vi "sub_Loop.vi"(0 "Input parameters":T2={"Measurement type"=enum."Test", "Sensor type"=enum."One channel", "Input file"="", "Output file"="test.txt", "Open after execution?"=FALSE, "Display channel"=0, "Voltage Delay (s)"=0.5, "Switch Delay (s)"=0.01, "VISA resource name source"="", "VISA resource name LCR"="", "Voltage Limit (V)"=1000.0, "Enable Voltage Auto Range (T:Enable)"=TRUE, "Voltage Manual Range (1.0)"=1.0, "Compliance  Level (uA)"=10.0} {"Voltage Limit (V)" format="%#_13g"; "Voltage Delay (s)" format="%#_13g"; "Switch Delay (s)" format="%#_13g"}, 2 "Current voltage":refnum<vi>, 3 "Voltages":refnum<vi>, 5 "Dynamic data 2":T1, 8 "Channels":refnum<vi>, 9 "Stop":refnum<vi>, 10 "Single channel":refnum<vi>, 11 "error in (no error)":errorcluster, 13 "Current channel":refnum<vi>) -> (4 "Input parameters":T2={"Measurement type"=enum."Test", "Sensor type"=enum."One channel", "Input file"="", "Output file"="test.txt", "Open after execution?"=FALSE, "Display channel"=0, "Voltage Delay (s)"=0.5, "Switch Delay (s)"=0.01, "VISA resource name source"="", "VISA resource name LCR"="", "Voltage Limit (V)"=1000.0, "Enable Voltage Auto Range (T:Enable)"=TRUE, "Voltage Manual Range (1.0)"=1.0, "Compliance  Level (uA)"=10.0} {"Voltage Limit (V)" format="%#_13g"; "Voltage Delay (s)" format="%#_13g"; "Switch Delay (s)" format="%#_13g"}, 6 "Dynamic data":T1, 15 "error out":errorcluster)   [LabVIEW 2015]
uses:
  Program Files (x86)/National Instruments/LabVIEW 2016/instr.lib/Keithley 24XX/Keithley 24XX.lvlib
  Program Files (x86)/National Instruments/LabVIEW 2016/instr.lib/Agilent 428X Series/Agilent 428X Series.lvlib
  Program Files (x86)/National Instruments/LabVIEW 2016/instr.lib/Keithley 24XX/Public/Data/Read (Single Point).vi
  Input_parameters.ctl
  Dynamic_data.ctl
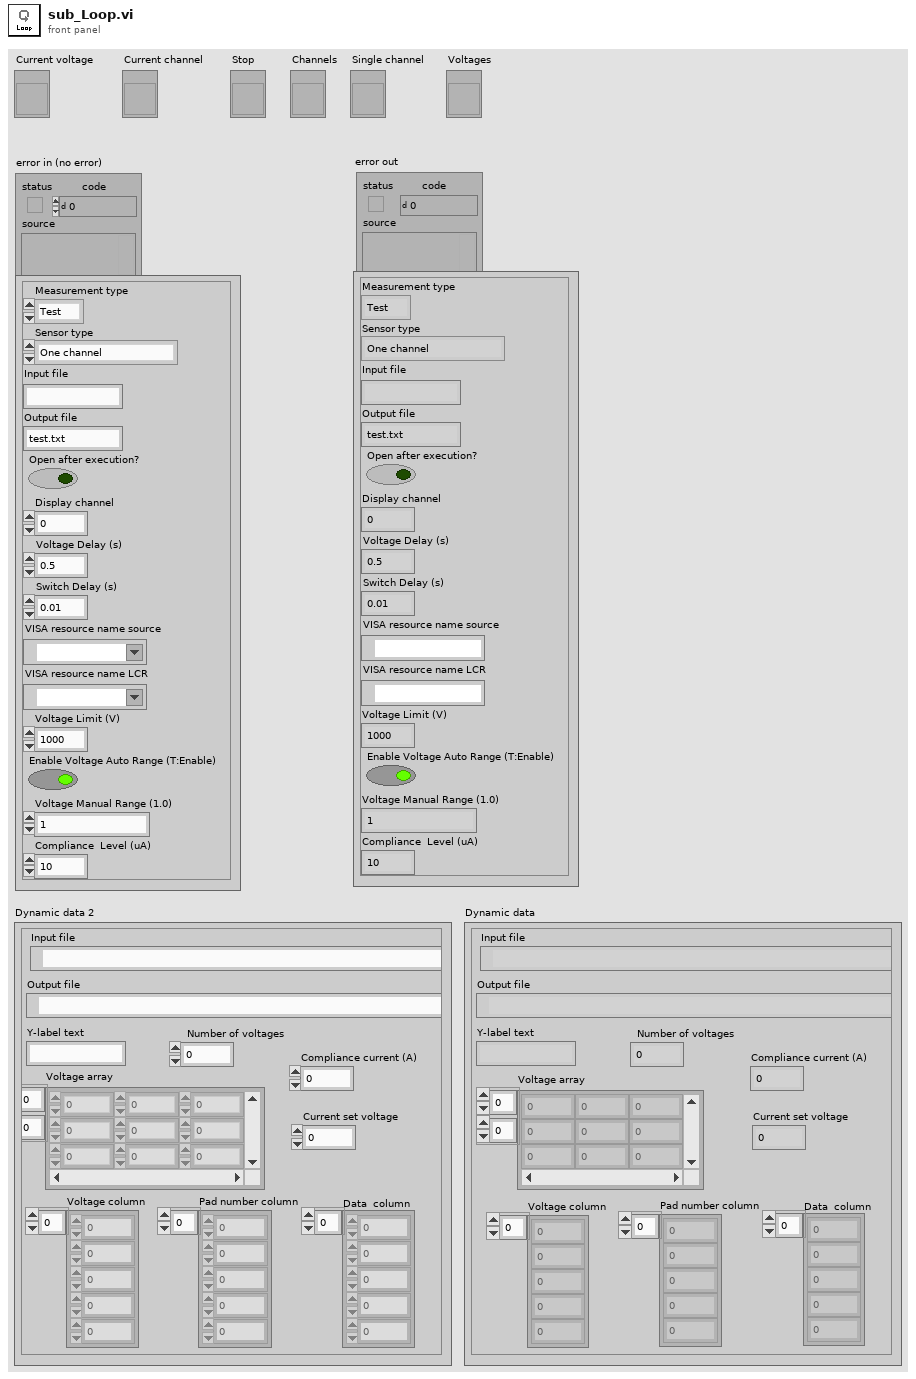
[diagram p1: front panel]
types:
  T1 = typedef "Dynamic_data.ctl" = cluster{"Input file":path, "Output file":path, "Y-label text":string, "Voltage array":dbl[][], "Current set voltage":dbl, "Voltage column":dbl[], "Pad number column":dbl[], "Data  column":dbl[], "Number of voltages":i32, "Compliance current (A)":dbl}
  T2 = typedef "Input_parameters.ctl" = cluster{"Measurement type":enum16{"IV", "CV", "Test"}, "Sensor type":enum16{"6''", "8''", "One channel"}, "Input file":string, "Output file":string, "Open after execution?":bool, "Display channel":i32, "Voltage Delay (s)":dbl, "Switch Delay (s)":dbl, "VISA resource name source":refnum<visa-resource-name>, "VISA resource name LCR":refnum<visa-resource-name>, "Voltage Limit (V)":dbl, "Enable Voltage Auto Range (T:Enable)":bool, "Voltage Manual Range (1.0)":dbl, "Compliance  Level (uA)":dbl}
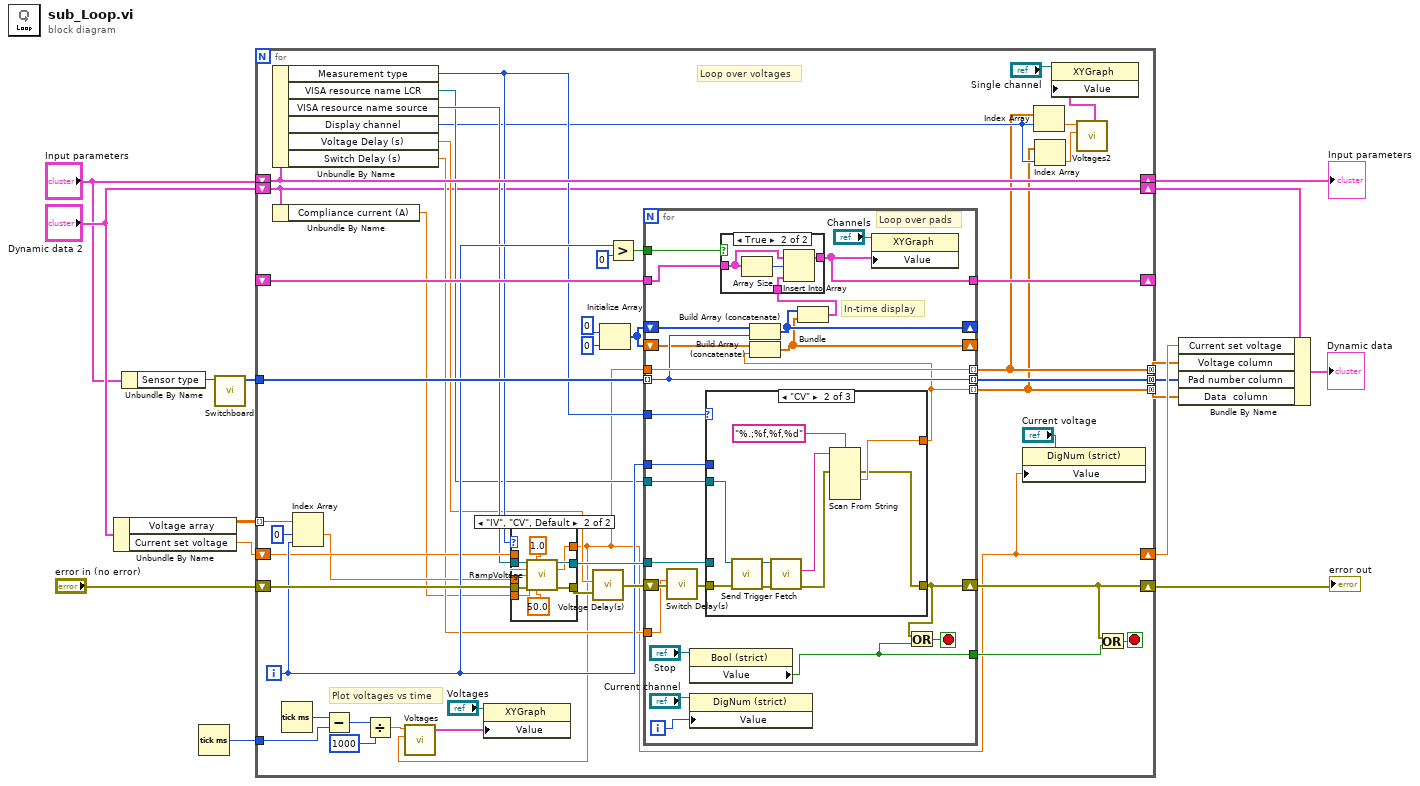
[diagram p0: block diagram]
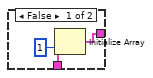
[diagram p3: hidden frame]
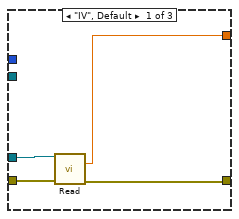
[diagram p4: hidden frame]
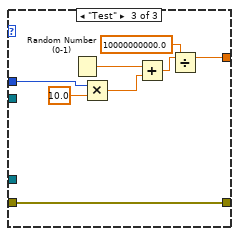
[diagram p5: hidden frame]
diagram:
  n1 = Unbundle By Name("Dynamic data 2") -> ("Voltage array"=w15:dbl[][], "Current set voltage"=w13:dbl)
  n2 = Unbundle By Name("Input parameters") -> ("Sensor type"=w16:enum16{"6''", "8''", "One channel"})
  n3 = Tick Count (ms)() -> (millisecond timer value=w1:u32)
  n4 = call "Switchboard.vi"("Sensor type"=w16) -> ("Output config"=w14:i32[])  [unwired: 10 in]
  n5 = for {
    tunnel: w15 -> [w61] mode=indexing
    tunnel: w14 -> [w59]
    tunnel: [w22] -> w11 mode=concatenating
    tunnel: [w21] -> w9 mode=concatenating
    tunnel: [w57] -> w10 mode=concatenating
    shift-right: [w43] -> w2
    shift-left: "error in (no error)" -> [w55]
    shift-right: [w51] -> _
    shift-left: _ -> [w50]
    shift-right: [w26] -> w12
    shift-left: w13 -> [w42]
    shift-right: [w40] -> w4
    shift-left: "Input parameters" -> [w40]
    shift-right: [w34] -> w8
    shift-left: "Dynamic data 2" -> [w34]
    tunnel: w1 -> [w27]
    i -> [w46]
    stop <- w44 stop-if-true
    # "Plot voltages vs time"
    # "Loop over voltages"
    n6 = Unbundle By Name(w40) -> ("Measurement type"=w39:enum16{"IV", "CV", "Test"}, "VISA resource name LCR"=w37:refnum<visa-resource-name>, "VISA resource name source"=w38:refnum<visa-resource-name>, "Display channel"=w23:i32, "Voltage Delay (s)"=w36:dbl, "Switch Delay (s)"=w35:dbl)
    n7 = Unbundle By Name(w34) -> ("Compliance current (A)"=w33:dbl)
    n8 = Tick Count (ms)() -> (millisecond timer value=w31:u32)
    n9 = Index Array(array=w61, index #1=0 ("index"), index #2=w46) -> (element #1=w41:dbl)  [unwired: 1 out]
    n10 = Subtract(x=w31, y=w27) -> (x-y=w30:u32)
    n11 = Divide(x=w30, y=u32 1000 ("x")) -> (x/y=w29:dbl)
    n12 = case shown="\"IV\", \"CV\", Default" w39 {
      tunnel: w38 -> [w64 w71]
      tunnel: w41 -> [w62 w70]
      tunnel: [w64 w73] -> w56
      tunnel: w55 -> [w63 w72]
      tunnel: [w63 w74] -> w54
      tunnel: w33 -> [_ w68]
      tunnel: w42 -> [_ w69]
      tunnel: [w62 w65] -> w26
      frame "Test" {
      }
      frame "IV", "CV", Default {
        n13 = call "RampVoltage.vi"("VISA resource name"=w71, "Delay (s)"=1.0, "Current voltage (V)"=w69, "Target voltage (V)"=w70, "Compliance Current (A)"=w68, "error in (no error)"=w72, "Step size (V)"=50.0) -> ("VISA resource name out"=w73:refnum<visa-resource-name>, "Current voltage out (V)"=w65:dbl, "error out"=w74:errorcluster)  [unwired: 6 in]
      }
    }
    n14 = call "Voltages"("Y Input"=w26, "X Input"=w29) -> ("XY Graph"=w17:cluster{"X":dbl[], "Y":dbl[]}[])  [unwired: 8 in, 1 out]
    n15 = property class="XYGraph"(reference="Voltages", "Value"=w17) -> ()  [unwired: 1 in, 2 out]
    n16 = call "Voltage Delay(s)"("error in (no error)"=w54, "Delay Time (s)"=w36) -> ("error out"=w53:errorcluster)  [unwired: 9 in]
    n17 = Initialize Array(0 ("dimension size"), 0 ("dimension size")) -> (w47:i32[])
    n18 = Greater?(x=w46, y=0) -> (0:w52:bool)
    n19 = for {
      tunnel: w59 -> [w95] mode=indexing
      tunnel: [w95] -> w57 mode=indexing
      tunnel: [w93] -> w21 mode=indexing
      tunnel: w26 -> [w99]
      tunnel: [w99] -> w22 mode=indexing
      tunnel: w56 -> [w97]
      tunnel: w39 -> [w98]
      shift-right: [w83] -> w43
      shift-left: w53 -> [w84]
      tunnel: w37 -> [w96]
      shift-right: [w91] -> _
      shift-left: w47 -> [w94]
      shift-right: [w90] -> _
      shift-left: w47 -> [w92]
      tunnel: w52 -> [w88]
      tunnel: w46 -> [w89]
      tunnel: w50 -> [w87]
      tunnel: [w75] -> w51
      tunnel: [w77] -> w45
      tunnel: w35 -> [w81]
      i -> [w79]
      stop <- w82 stop-if-true
      # "In-time display"
      # "Loop over pads"
      n20 = call "Switch Delay(s)"("error in (no error)"=w84, "Delay Time (s)"=w81) -> ("error out"=w85:errorcluster)  [unwired: 9 in]
      n21 = property class="Bool (strict)"(reference="Stop") -> ("Value"=w77:bool)  [unwired: 1 in, 2 out]
      n22 = property on="Property Node" class="DigNum (strict)"(reference="Current channel", "Value"=w79) -> ()  [unwired: 1 in, 2 out]
      n23 = case shown="\"CV\"" w98 {
        tunnel: [w110 w113 w121] -> w93
        tunnel: w97 -> [w108 _ _]
        tunnel: w85 -> [w109 w116 w127]
        tunnel: [w107 w111 w127] -> w83
        tunnel: w96 -> [_ w117 _]
        tunnel: w89 -> [_ _ w122]
        frame "IV", Default {
          n24 = call-poly "Read.vi"("VISA resource name"=w108, "error in (no error)"=w109) -> ("Current"=w110:sgl, "error out"=w107:errorcluster)  [unwired: 7 in, 5 out]
        }
        frame "CV" {
          n25 = call "Send Trigger.vi"("error in (no error)"=w116, "VISA resource name"=w117) -> ("error out"=w118:errorcluster, "VISA resource name out"=w119:refnum<visa-resource-name>)  [unwired: 8 in]
          n26 = call "Fetch.vi"("error in (no error)"=w118, "VISA resource name"=w119) -> ("error out"=w112:errorcluster, "Returned Data"=w114:string)  [unwired: 7 in, 1 out]
          n27 = Scan From String(format string="%.;%f,%f,%d", input string=w114, error in=w112) -> (error out=w111:errorcluster, output 1=w113:dbl)  [unwired: 6 in, 2 out]
        }
        frame "Test" {
          n28 = Random Number (0-1)() -> (number: 0 to 1=w126:dbl)
          n29 = Multiply(x=w122, y=10.0) -> (x*y=w123:dbl)
          n30 = Add(x=w126, y=w123) -> (x+y=w125:dbl)
          n31 = Divide(x=w125, y=10000000000.0) -> (x/y=w121:dbl)
        }
      }
      n32 = Build Array (concatenate)(w94, w95) -> (w91:i32[])
      n33 = Build Array (concatenate)(w92, w93) -> (w90:dbl[])
      n34 = Bundle(w91, w90) -> (w86:cluster{i32[], dbl[]})  [unwired: 1 out]
      n35 = case shown="True" w88 {
        tunnel: w87 -> [_ w105]
        tunnel: [w100 w104] -> w75
        tunnel: w86 -> [w101 w103]
        frame False {
          n36 = Initialize Array(w101, 1 ("dimension size")) -> (w100:cluster{i32[], dbl[]}[])
        }
        frame True {
          n37 = Array Size(array=w105) -> (size(s)=w106:i32)
          n38 = Insert Into Array(array=w105, index=w106, new element=w103) -> (w104:cluster{i32[], dbl[]}[])
        }
      }
      n39 = property class="XYGraph"(reference="Channels", "Value"=w75) -> ()  [unwired: 1 in, 2 out]
      n40 = Or(x=w83, y=w77) -> (x .or. y?=w82:bool)
    }
    n41 = property class="DigNum (strict)"(reference="Current voltage", "Value"=w26) -> ()  [unwired: 1 in, 2 out]
    n42 = Index Array(array=w22, index=w23) -> (element=w25:dbl)
    n43 = Index Array(array=w21, index=w23) -> (element=w24:dbl)
    n44 = call "Voltages2"("Y Input"=w24, "X Input"=w25) -> ("XY Graph"=w19:cluster{"X":dbl[], "Y":dbl[]}[])  [unwired: 8 in, 1 out]
    n45 = property class="XYGraph"(reference="Single channel", "Value"=w19) -> ()  [unwired: 1 in, 2 out]
    n46 = Or(x=w43, y=w45) -> (x .or. y?=w44:bool)
  }
  "error out" <- w2
  "Input parameters" <- w4
  n47 = Bundle By Name(cluster=w8, "Current set voltage"=w12, "Voltage column"=w11, "Pad number column"=w10, "Data  column"=w9) -> (→"Dynamic data":T1)
